vi "RWA_Insert Section String into File String.vi"(9 "Section Name":string, 10 "Strings[]":string[](array[string]), 11 "File String":string) -> (2 "Section Replaced Out":bool, 3 "File String Out":string)   [LabVIEW 2020]
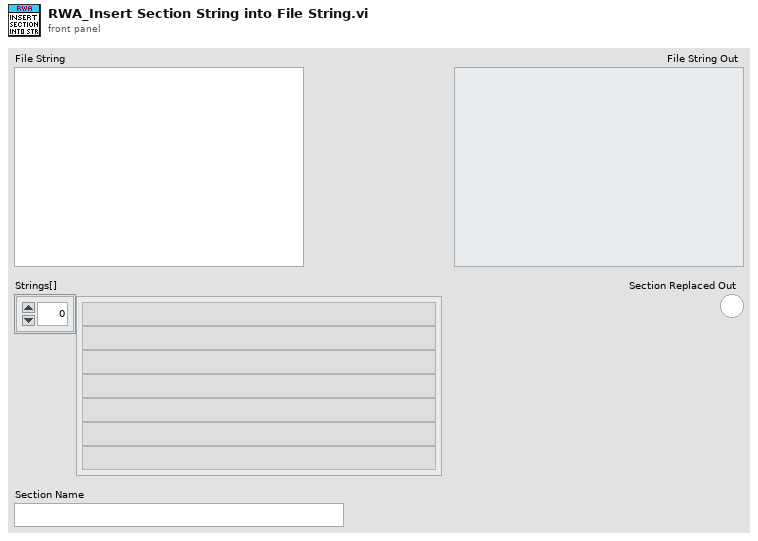
[diagram p1: front panel]
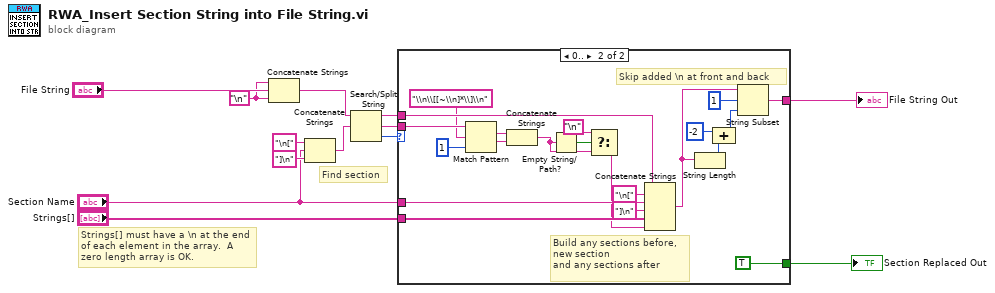
[diagram p0: block diagram]
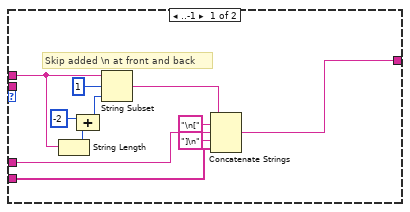
[diagram p2: hidden frame]
diagram:
  w5 = "\n"
  # "Strings[] must have a \\n at the end of each element in the array.  A zero length array is OK."
  # "Find section"
  n1 = Concatenate Strings(w5, "File String", w5) -> (w6:string)
  n2 = Concatenate Strings("\n[" ("string"), "Section Name", "]\n" ("string")) -> (w7:string)
  n3 = Search/Split String(string=w6, search string/char (-)=w7) -> (substring before match=w8:string, match + rest of string=w9:string, offset of match=w11:i32)  [unwired: 1 in]
  n4 = case shown="0.." w11 {
    tunnel: "Section Name" -> [w22 w45]
    tunnel: "Strings[]" -> [w21 w44]
    tunnel: w8 -> [w15 w43]
    tunnel: [w20 w41] -> w13
    tunnel: w9 -> [_ w36]
    tunnel: [_ TRUE] -> w12
    frame ..-1 {
      # "Skip added \\n at front and back"
      n5 = String Length(string=w15) -> (length=w18:i32)
      n6 = Compound Arithmetic op=ADD(-2 ("value"), w18) -> (w17:i32)
      n7 = String Subset(string=w15, offset (0)=1, length (rest)=w17) -> (substring=w14:string)
      n8 = Concatenate Strings(w14, "\n[" ("string"), w22, "]\n" ("string"), w21) -> (w20:string)
    }
    frame 0.. {
      # "Build any sections before,\nnew section\nand any sections after"
      # "Skip added \\n at front and back"
      n9 = Match Pattern(string=w36, regular expression="\\n\\[[~\\n]*\\]\\n", offset (0)=1) -> (match substring=w30:string, after substring=w29:string)  [unwired: 2 out]
      n10 = Concatenate Strings(w30, w29) -> (w27:string)
      n11 = Empty String/Path?(string/path=w27) -> (empty?=w32:bool)
      n12 = Select(t="\n", s=w32, f=w27) -> (s? t:f=w31:string)
      n13 = Concatenate Strings(w43, "\n[" ("string"), w45, "]\n" ("string"), w44, w31) -> (w42:string)
      n14 = String Length(string=w42) -> (length=w39:i32)
      n15 = Compound Arithmetic op=ADD(-2 ("value"), w39) -> (w38:i32)
      n16 = String Subset(string=w42, offset (0)=1, length (rest)=w38) -> (substring=w41:string)
    }
  }
  "File String Out" <- w13
  "Section Replaced Out" <- w12
